vi "taskmgr.vi"() -> ()   [LabVIEW 2009]
uses:
  main states.ctl
  <vilib>/Platform/TimedLoop/XDataNode/XDataNode.xnode
  <vilib>/Platform/TimedLoop/XDataNode/loadlvalarms.vi
  <vilib>/Platform/TimedLoop/XDataNode/timing_clust.ctl
  <vilib>/Platform/TimedLoop/XDataNode/nitl_modes.ctl
  <vilib>/Platform/TimedLoop/XDataNode/wakeup.ctl
  <vilib>/Platform/TimedLoop/XDataNode/XDNodeRunTimeDep.lvlib
panel:
  out "Execution:State":T1(ring)
  out "Numeric":i32
  out "Iteration Duration":i64
  out "elements":T2[](array[typedef])
  out "Current State":T2
  in  "Start/Stop Counter":bool
  in  "stop":bool
  out "Counter on?":bool
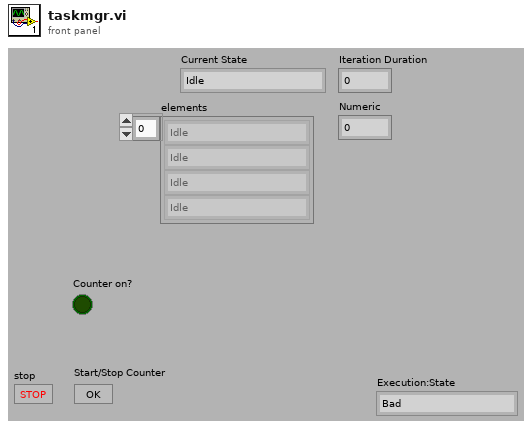
[diagram p1: front panel]
types:
  T1 = enum32{"Bad", "Idle", "Run top level", "Running"}
  T2 = typedef "main states.ctl" = enum16{"Idle", "Set Counter Period", "Toggle Counter", "Stop"}
  T3 = typedef "XDNodeRunTimeDep.lvlib/timing_clust.ctl" = cluster{"Expected End [f-1]":u64, "Actual End [f-1]":u64, "Finished Late? [f-1]":bool, "Expected End [i-1]":u64, "Actual End [i-1]":u64, "Finished Late? [i-1]":bool, "Expected Start [i]":u64, "Actual Start [i]":u64, "Expected Start [f]":u64, "Actual Start [f]":u64, "Source Name":string, "Structure Name":string, "Period":i64, "Deadline":i64, "Offset":i64, "Start":i64, "Priority":i32, "Timeout":i32, "Mode":T4, "Wakeup Reason":T5, "Error":errorcluster, "Source Type":string, "Secondary Source Type":string, "Global End Time":u64, "Global Start Time":u64, "Frame Duration":u64, "Iteration Duration":u64, "Assigned CPU":i32, "I/O Scan Engine Mode":u32}
  T4 = typedef "XDNodeRunTimeDep.lvlib/nitl_modes.ctl" = enum32{"No Change", "Process missed periods, maintain original phase", "Discard missed periods, maintain original phase", "Process missed periods, ignore original phase", "Discard missed periods, ignore original phase"}
  T5 = typedef "XDNodeRunTimeDep.lvlib/wakeup.ctl" = enum32{"Normal", "Aborted", "Asynchronous wakeup", "Timing source error", "Timed loop error", "Timeout"}
  T6 = typedef "UDP Base.ctl" = cluster{"UDP Session":refnum<k16>, "UDP Socket Params":T7}
  T7 = typedef "UDP Socket Params.ctl" = cluster{"Local Port":u16, "Read Timeout":i32, "Write Timeout":i32}
  T8 = typedef "UDP Network Location.ctl" = cluster{"IP Address":string, "Port":u16}
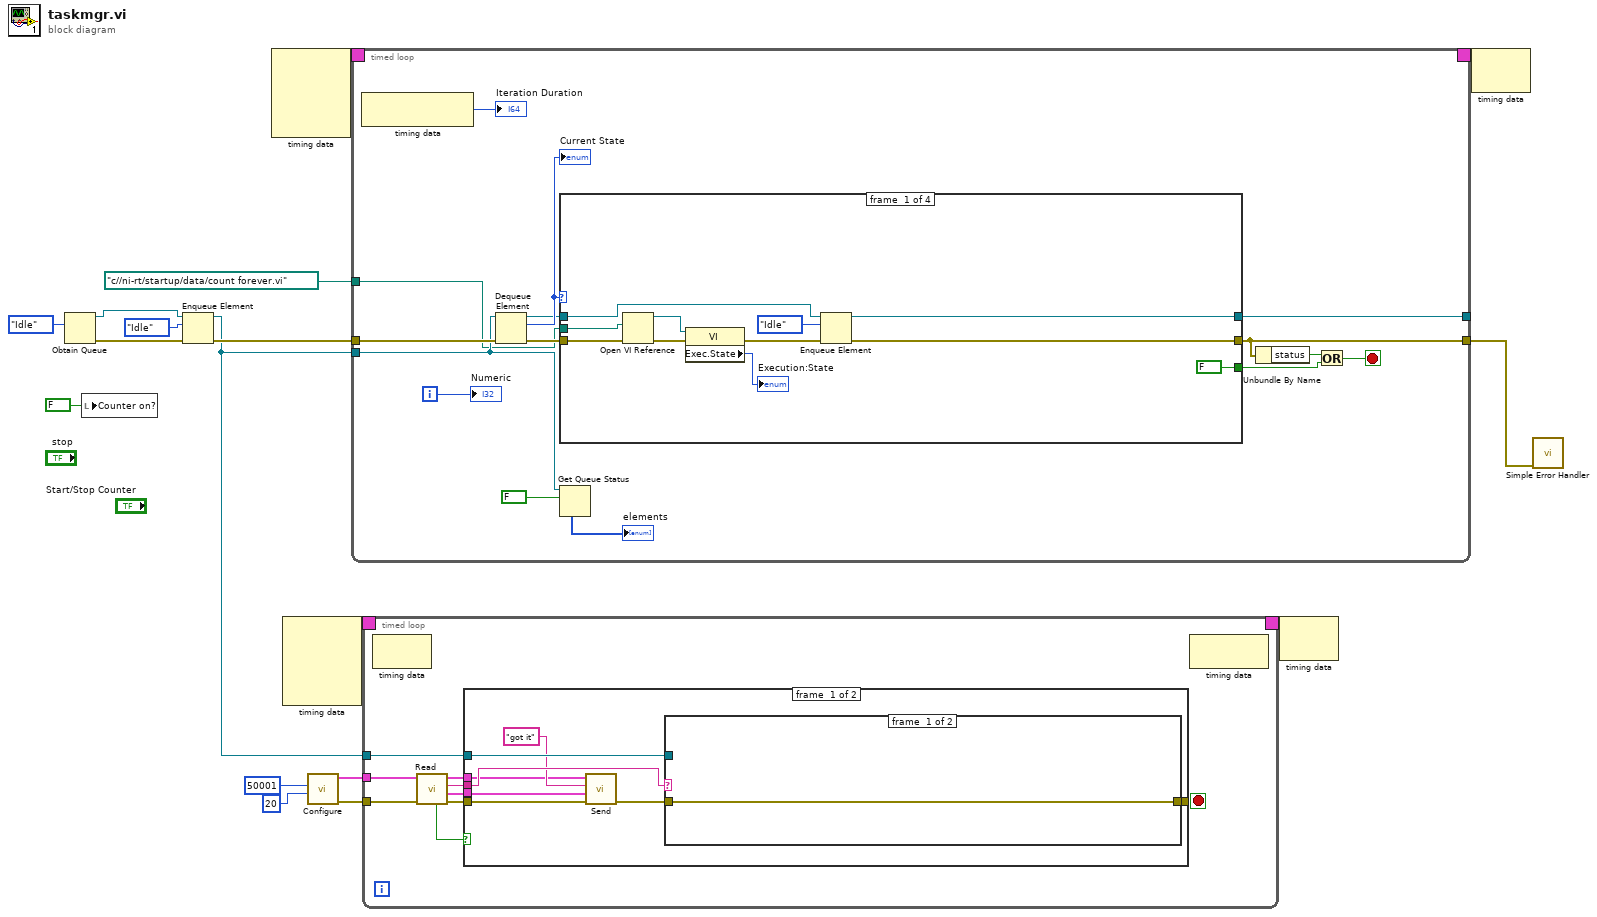
[diagram p0: block diagram]
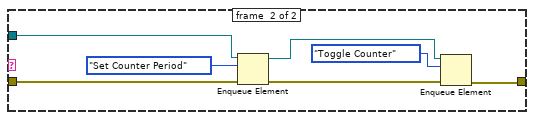
[diagram p2: hidden frame]
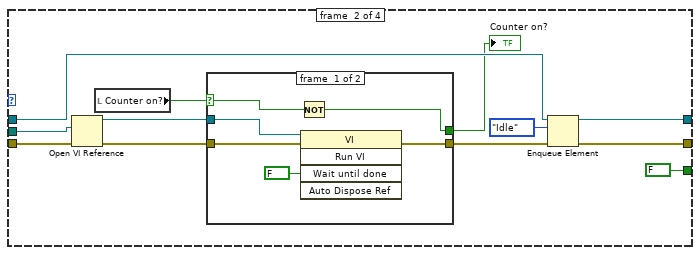
[diagram p4: hidden frame]
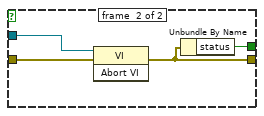
[diagram p5: hidden frame]
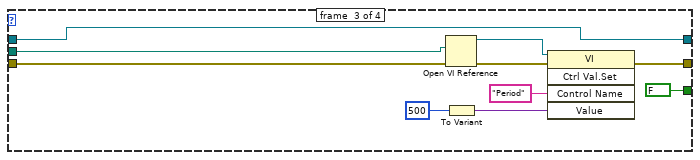
[diagram p6: hidden frame]
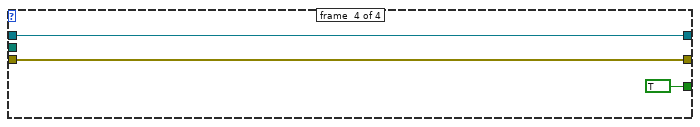
[diagram p7: hidden frame]
diagram:
  n1 = Obtain Queue(element data type=main_states."Idle" ("States")) -> (queue out=w14:refnum<queue>, error out=w13:errorcluster)  [unwired: 4 in, 1 out]
  n2 = local write "Counter on?"(FALSE ("Counter on?")) -> ()
  n3 = Enqueue Element(queue=w14, element=main_states."Idle", error in (no error)=w13) -> (queue out=w4:refnum<queue>, error out=w12:errorcluster)  [unwired: 1 in, 1 out]
  n4 = node-c288() -> (w11:T3)  [unwired: 4 in]
  n5 = node-c288() -> (w8:T3)  [unwired: 4 in]
  n6 = call "Configure.vi"("Read Timeout"=20, "Local Port"=u16 50001) -> ("error out"=w5:errorcluster, "UDP Base out"=w6:T6)  [unwired: 8 in]
  n7 = timed-loop {
    tunnel: w4 -> [w20]
    tunnel: w12 -> [w31]
    tunnel: [w27] -> _
    tunnel: [w26] -> w16
    timing: w11 -> [_]
    timing-out: [_] -> w10
    tunnel: path "c://ni-rt/startup/data/count forever.vi" ("base path") -> [w18]
    i -> [w19]
    stop <- w28 stop-if-true
    n8 = node-c288() -> (→"Iteration Duration":i64)  [unwired: 1 in]
    n9 = Dequeue Element(queue=w20, error in (no error)=w31) -> (queue out=w24:refnum<queue>, element=w32:T2, error out=w30:errorcluster)  [unwired: 1 in, 1 out]
    "Current State" <- w32
    n10 = case shown="\"Set Counter Period\"" w32 {
      tunnel: w30 -> [w38 w48 w77 w80]
      tunnel: w24 -> [w45 w56 w68 w79]
      tunnel: [w44 w55 w68 w79] -> w27
      tunnel: [w43 w53 w70 w80] -> w26
      tunnel: [FALSE ("status") FALSE ("status") FALSE ("status") TRUE ("status")] -> w25
      tunnel: w18 -> [w40 w49 w76 _]
      frame #0 {
        n11 = Open VI Reference(vi path=w40, error in (no error)=w38) -> (vi reference=w36:refnum<vi>, error out=w39:errorcluster)  [unwired: 4 in]
        n12 = property class="VI"(reference=w36, error in=w39) -> (error out=w37:errorcluster, "Exec.State"=→"Execution:State":T1)  [unwired: 1 out]
        n13 = Enqueue Element(queue=w45, element=main_states."Idle", error in (no error)=w37) -> (queue out=w44:refnum<queue>, error out=w43:errorcluster)  [unwired: 1 in, 1 out]
      }
      frame #1 {
        n14 = Open VI Reference(vi path=w49, error in (no error)=w48) -> (vi reference=w46:refnum<vi>, error out=w47:errorcluster)  [unwired: 4 in]
        n15 = local read "Counter on?"() -> (w52:bool)
        n16 = case shown="False" w52 {
          selector: w52 -> [w63 _]
          tunnel: [w60 w65] -> w54
          tunnel: [w62 w64] -> w51
          tunnel: w47 -> [w59 w66]
          tunnel: w46 -> [w58 w67]
          frame #0 {
            n17 = Not(x=w63) -> (.not. x?=w62:bool)
            n18 = invoke class="VI" method="Run VI"(reference=w58, error in=w59, "Wait until done"=FALSE ("Wait Until Done")) -> (error out=w60:errorcluster)  [unwired: 2 in, 4 out]
          }
          frame #1 {
            n19 = invoke class="VI" method="Abort VI"(reference=w67, error in=w66) -> (error out=w65:errorcluster)  [unwired: 1 in, 2 out]
            n20 = Unbundle By Name(w65) -> ("status"=w64:bool)
          }
        }
        "Counter on?" <- w51
        n21 = Enqueue Element(queue=w56, element=main_states."Idle", error in (no error)=w54) -> (queue out=w55:refnum<queue>, error out=w53:errorcluster)  [unwired: 1 in, 1 out]
      }
      frame #2 {
        n22 = Open VI Reference(vi path=w76, error in (no error)=w77) -> (vi reference=w74:refnum<vi>, error out=w75:errorcluster)  [unwired: 4 in]
        n23 = To Variant(anything=i64 500 ("Counter Period")) -> (Variant=w72:variant)
        n24 = invoke class="VI" method="Ctrl Val.Set"(reference=w74, error in=w75, "Control Name"="Period", "Value"=w72) -> (error out=w70:errorcluster)  [unwired: 1 in, 4 out]
      }
      frame #3 {
      }
    }
    n25 = Get Queue Status(queue=w20, return elements? (F)=FALSE) -> (elements=→"elements":T2[])  [unwired: 1 in, 7 out]
    n26 = Unbundle By Name(w26) -> ("status"=w29:bool)
    n27 = Or(x=w29, y=w25) -> (x .or. y?=w28:bool)
    "Numeric" <- w19
  }
  n28 = timed-loop {
    timing: w8 -> [_]
    timing-out: [_] -> w7
    tunnel: w6 -> [w88]
    tunnel: w5 -> [w89]
    tunnel: w4 -> [w86]
    stop <- _ stop-if-true
    n29 = node-c288() -> ()  [unwired: 1 in, 1 out]
    n30 = call "Read.vi"("error in (no error)"=w89, "UDP Base in"=w88) -> ("error out"=w85:errorcluster, "Network Location"=w83:T8, "Receive Data"=w87:string, "UDP Base out"=w82:T6, "Timeout"=w84:bool)  [unwired: 4 in, 1 out]
    n31 = case shown="False" w84 {
      tunnel: w87 -> [w97 _]
      tunnel: w86 -> [w96 _]
      tunnel: w85 -> [w94 w106]
      tunnel: [w95 w106] -> _
      tunnel: w83 -> [w92 _]
      tunnel: w82 -> [w91 _]
      frame #0 {
        n32 = call "Send.vi"("error in (no error)"=w94, "Destination Location"=w92, "Send Data"="got it", "UDP Base in"=w91) -> ("error out"=w90:errorcluster)  [unwired: 5 in, 2 out]
        n33 = case shown="\"toggle\"" w97 {
          tunnel: w96 -> [_ w101]
          tunnel: w90 -> [w98 w102]
          tunnel: [w98 w99] -> w95
          frame #0 {
          }
          frame #1 {
            n34 = Enqueue Element(queue=w101, element=main_states."Set Counter Period", error in (no error)=w102) -> (queue out=w100:refnum<queue>, error out=w103:errorcluster)  [unwired: 1 in, 1 out]
            n35 = Enqueue Element(queue=w100, element=main_states."Toggle Counter", error in (no error)=w103) -> (error out=w99:errorcluster)  [unwired: 1 in, 2 out]
          }
        }
      }
      frame #1 {
      }
    }
    n36 = node-c288() -> ()  [unwired: 1 in, 1 out]
  }
  n37 = node-c288(w7) -> ()  [unwired: 1 out]
  n38 = node-c288(w10) -> ()  [unwired: 1 out]
  n39 = call <vilib>:"Simple Error Handler.vi"("error in (no error)"=w16) -> ()  [unwired: 4 in, 5 out]
